vi "I(V)_MFLI_PK_v4.0_measureR.vi"() -> ()   [LabVIEW 2016]
uses:
  Labview Drivers/MFLI/LabOneLabVIEW-22.02.26577/LabOneLabVIEW-22.02.26577/Zurich Instruments LabOne/Public/Data/ziTypeDemodSampleSingle.ctl
  Labview Drivers/MFLI/LabOneLabVIEW-22.02.26577/LabOneLabVIEW-22.02.26577/Zurich Instruments LabOne/Public/Configure/ziSetValueDouble.vi
  Labview Drivers/MFLI/LabOneLabVIEW-22.02.26577/LabOneLabVIEW-22.02.26577/Zurich Instruments LabOne/Public/Configure/ziGetValueDemodSampleEx.vi
  Labview Drivers/MFLI/LabOneLabVIEW-22.02.26577/LabOneLabVIEW-22.02.26577/Zurich Instruments LabOne/Zurich Instruments LabOne.lvlib
panel:
  out "Set Voltage(V)":dbl format="%#_13g"
  out "Time(s)":dbl format="%#_13g"
  out "Demod Sample Out 2":T1={"Timestamps (ticks)"=34359738372, "X (Vrms)"=8.366245757779461e-285, "Y (Vrms)"=1.0096057436928657e-284, "Osc Phase (deg)"=1.69759663376e-313, "Freq (Hz)"=2.607691286315397e-191, "DIO"=4, "AuxIn0 (V)"=0.0, "AuxIn1 (V)"=1.6954746369817e-311, "Trigger"=16}
  out "Demod Sample Out":T1={"Timestamps (ticks)"=34359738372, "X (Vrms)"=8.366245757779461e-285, "Y (Vrms)"=1.0096057436928657e-284, "Osc Phase (deg)"=1.69759663376e-313, "Freq (Hz)"=2.607691286315397e-191, "DIO"=4, "AuxIn0 (V)"=0.0, "AuxIn1 (V)"=1.6954746369817e-311, "Trigger"=16}
  in  "MFLI Current source/Voltage reader":string="DEV4382"
  out "Imeas (A)":dbl=2.528615115e-315
  out "Vmeas (V)":dbl=nan
  in  "Folder":path=path "D:/Pranava/Data/Mn3Ge/MA1141"
  in  "wait (ms) [Should be > TC]":u32=1000
  out "I vs V":cluster{dbl, "Field Reading":dbl}[](graph)=[{nan, "Field Reading"=3.54694038e-315}, {nan, "Field Reading"=2.528615115e-315}]
  out "data":dbl[](array[numeric])=[nan, 2.528615115e-315, 0.0001]
  in  "Step":dbl[](array[numeric])=[0.05, 0.05, 0.05] min=-3000.0 max=3000.0 format="%.1e"
  in  "To":dbl[](array[numeric])=[7.0, -7.0, 0.0] min=-3000.0 max=3000.0 format="%.1e"
  in  "From":dbl[](array[numeric])=[0.0, 7.0, -7.0] min=-3000.0 max=3000.0 format="%.1e"
  in  "file name":string="002_MA1141_Mn3Ge(1120)IV_VdP_4K_slow"
  out "File path":path=path "D:/Pranava/Data/Mn3Ge/MA1141/002_MA1141_Mn3Ge(1120)IV_VdP_4K_slow.dat"
  # ".dat"
  # "Set MFLI Voltage output (V)"
types:
  T1 = typedef "Zurich Instruments LabOne.lvlib/ziTypeDemodSampleSingle.ctl" = cluster{"Timestamps (ticks)":u64, "X (Vrms)":dbl, "Y (Vrms)":dbl, "Osc Phase (deg)":dbl, "Freq (Hz)":dbl, "DIO":u32, "AuxIn0 (V)":dbl, "AuxIn1 (V)":dbl, "Trigger":u32}
  T2 = enum16{"open", "replace", "create", "open or create", "replace or create", "replace or create with confirmation"}
  T3 = typedef "Zurich Instruments LabOne.lvlib/ziTypeHandle.ctl" = cluster{"handleValid":bool, "Conn":u64, "Path Prefix":string, "Handle":u64, "Connected":bool, "Clockbase(s)":dbl}
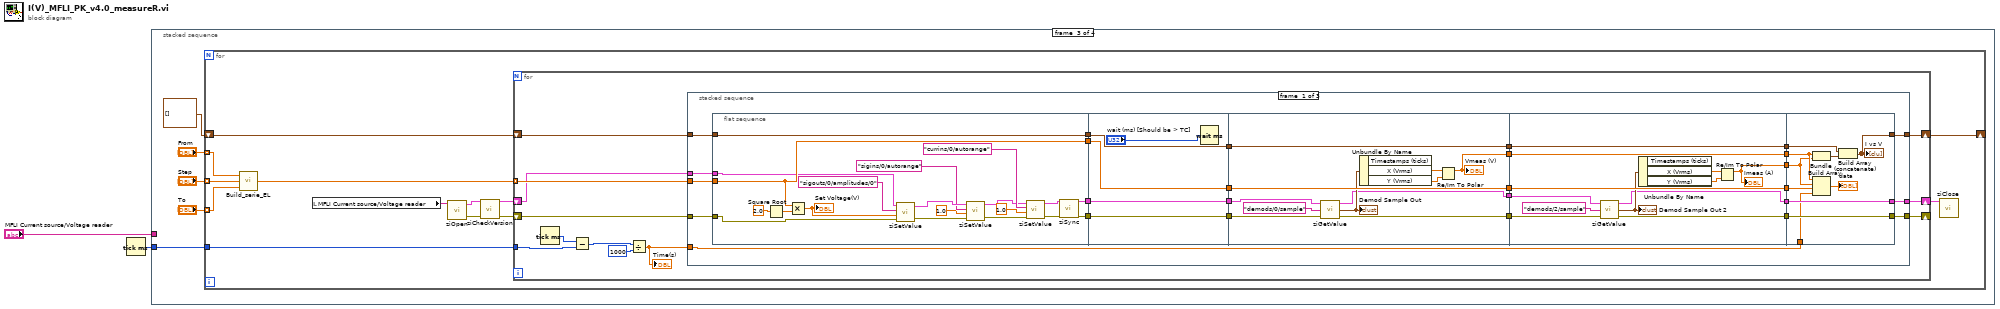
[diagram p0: block diagram]
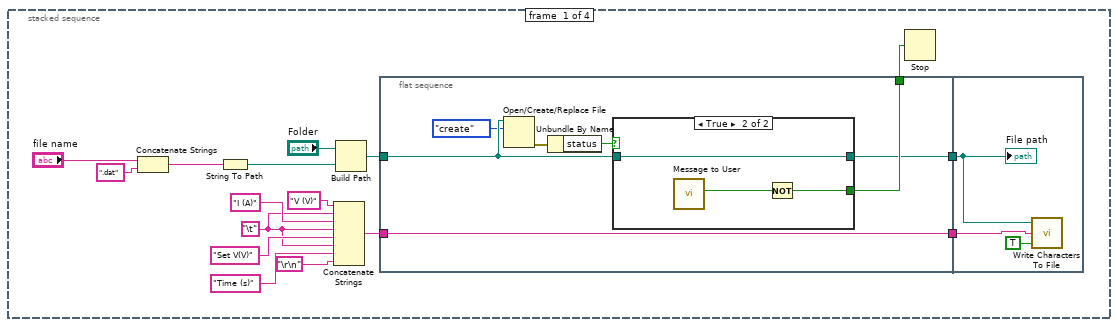
[diagram p2: hidden frame]
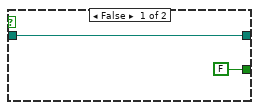
[diagram p3: hidden frame]
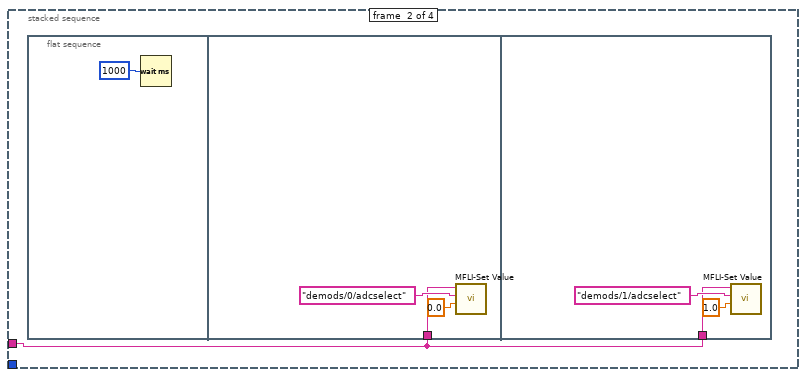
[diagram p4: hidden frame]
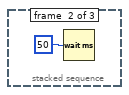
[diagram p5: hidden frame]
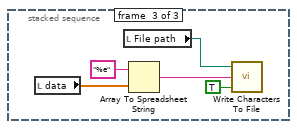
[diagram p6: hidden frame]
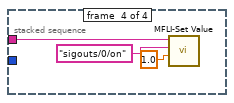
[diagram p7: hidden frame]
diagram:
  n1 = Tick Count (ms)() -> (millisecond timer value=w1:u32)
  n2 = stacked-sequence {
    tunnel: "MFLI Current source/Voltage reader" -> [_ w34 _ w163]
    tunnel: w1 -> [_ _ w42 _]
    frame #0 {
      w4 = "\t"
      n3 = Concatenate Strings("file name", ".dat" ("string")) -> (w15:string)
      n4 = String To Path(string=w15) -> (path=w7:path)
      n5 = Concatenate Strings("V (V)" ("string"), w4, "I (A)" ("string"), w4, "Set V(V)" ("string"), w4, "Time (s)", "\r\n") -> (w16:string)
      n6 = Build Path(base path="Folder", name or relative path=w7) -> (appended path=w6:path)
      n7 = flat-sequence {
        tunnel: w6 -> [w22]
        tunnel: w16 -> [w25]
        tunnel: [w25] -> w18
        tunnel: [w24] -> w13
        tunnel: [w23] -> w17
        tunnel: w18 -> [w32]
        tunnel: w17 -> [w31]
        frame #0 {
          n8 = Open/Create/Replace File(file path (use dialog)=w22, operation (0:open)=T2."create") -> (error out=w21:errorcluster)  [unwired: 4 in, 2 out]
          n9 = Unbundle By Name(w21) -> ("status"=w19:bool)
          n10 = case shown="True" w19 {
            tunnel: [FALSE ("Yes") w29] -> w24
            tunnel: [w26 w28] -> w23
            tunnel: w22 -> [w26 w28]
            frame False {
            }
            frame True {
              n11 = call "Message to User"() -> ("Yes"=w30:bool)  [unwired: 10 in, 1 out]
              n12 = Not(x=w30) -> (.not. x?=w29:bool)
            }
          }
        }
        frame #1 {
          n13 = call <vilib>:"Write Characters To File.vi"("append to file? (new file:F)"=TRUE, "character string"=w32, "file path (dialog if empty)"=w31) -> ()  [unwired: 2 in, 1 out]
          "File path" <- w31
        }
      }
      n14 = Stop(stop? (T)=w13) -> ()
    }
    frame #1 {
      n15 = flat-sequence {
        tunnel: w34 -> [w36]
        tunnel: w34 -> [w39]
        frame #0 {
          n16 = Wait (ms)(milliseconds to wait=u32 1000) -> ()  [unwired: 1 out]
        }
        frame #1 {
          n17 = call "MFLI-Set Value.vi"("Value"=0.0, "Path"="demods/0/adcselect", "MFLI Current source/Voltage reader"=w36) -> ()  [unwired: 9 in]
        }
        frame #2 {
          n18 = call "MFLI-Set Value.vi"("Value"=1.0, "Path"="demods/1/adcselect", "MFLI Current source/Voltage reader"=w39) -> ()  [unwired: 9 in]
        }
      }
    }
    frame #2 {
      n19 = for {
        tunnel: "From" -> [w56] mode=indexing
        tunnel: "To" -> [w55] mode=indexing
        tunnel: "Step" -> [w54] mode=indexing
        shift-right: [w58] -> _
        shift-left: cluster{dbl, "Field Reading":dbl}[] [] -> [w59]
        tunnel: w42 -> [w47]
        n20 = call "Build_serie_EL.vi"("end value"=w55, "increment"=w54, "start value"=w56) -> ("output array"=w57:dbl[])
        n21 = local read "MFLI Current source/Voltage reader"() -> (w53:string)
        n22 = call "ziOpen.vi"("Address"=w53) -> ("Error Out"=w52:errorcluster, "HandleOut"=w51:T3)  [unwired: 3 in, 1 out]
        n23 = call "ziCheckVersion.vi"("Handle In"=w51, "Error In"=w52) -> ("Handle Out"=w50:T3, "Error Out"=w48:errorcluster)  [unwired: 11 in, 1 out]
        n24 = for {
          tunnel: w57 -> [w71] mode=indexing
          shift-right: [w69] -> w58
          shift-left: w59 -> [w70]
          shift-right: [w66] -> w49
          shift-left: w50 -> [w68]
          shift-right: [w65] -> _
          shift-left: w48 -> [w67]
          tunnel: w47 -> [w61]
          n25 = Tick Count (ms)() -> (millisecond timer value=w62:u32)
          n26 = Subtract(x=w62, y=w61) -> (x-y=w63:u32)
          n27 = Divide(x=w63, y=1000) -> (x/y=w60:dbl)
          "Time(s)" <- w60
          n28 = stacked-sequence {
            tunnel: w71 -> [w96 _ _]
            tunnel: w70 -> [w97 _ _]
            tunnel: [w98 _ _] -> w69
            tunnel: w68 -> [w87 _ _]
            tunnel: w67 -> [w86 _ _]
            tunnel: [w76 _ _] -> w66
            tunnel: [w75 _ _] -> w65
            tunnel: w60 -> [w72 _ _]
            frame #0 {
              n29 = flat-sequence {
                tunnel: [w118] -> w93
                tunnel: [w117] -> w92
                tunnel: w96 -> [w117]
                tunnel: w97 -> [w118]
                tunnel: [w100] -> w89
                tunnel: [w101] -> w88
                tunnel: w87 -> [w103]
                tunnel: w86 -> [w102]
                tunnel: w93 -> [w123]
                tunnel: [w123] -> w95
                tunnel: w92 -> [w122]
                tunnel: [w122] -> w94
                tunnel: [w120] -> w91
                tunnel: [w119] -> w90
                tunnel: w89 -> [w119]
                tunnel: w88 -> [w120]
                tunnel: [w124] -> w85
                tunnel: [w134] -> w83
                tunnel: [w133] -> w81
                tunnel: w90 -> [w130]
                tunnel: w91 -> [w129]
                tunnel: w95 -> [w134]
                tunnel: w94 -> [w133]
                tunnel: [w128] -> w79
                tunnel: [w127] -> w78
                tunnel: w85 -> [w138]
                tunnel: [w138] -> w84
                tunnel: w83 -> [w146]
                tunnel: [w146] -> w82
                tunnel: w81 -> [w145]
                tunnel: [w145] -> w80
                tunnel: w79 -> [w142]
                tunnel: w78 -> [w141]
                tunnel: [w140] -> w77
                tunnel: [w139] -> w74
                tunnel: [w135] -> w73
                tunnel: w84 -> [w155]
                tunnel: [w154] -> w98
                tunnel: w82 -> [w153]
                tunnel: w80 -> [w152]
                tunnel: [w151] -> w76
                tunnel: w77 -> [w151]
                tunnel: [w150] -> w75
                tunnel: w74 -> [w150]
                tunnel: w73 -> [w149]
                tunnel: w72 -> [w147]
                frame #0 {
                  n30 = Square Root(x=2.0) -> (sqrt(x)=w116:dbl)
                  n31 = Multiply(x=w117, y=w116) -> (x*y=w99:dbl)
                  "Set Voltage(V)" <- w99
                  n32 = call-poly "ziSetValue.vi"("Error In"=w102, "Value"=w99, "Path"="sigouts/0/amplitudes/0", "Handle In"=w103) -> ("Error Out"=w110:errorcluster, "Handle Out"=w113:T3)  [unwired: 1 in]
                  n33 = call-poly "ziSetValue.vi"("Error In"=w110, "Value"=1.0, "Path"="sigins/0/autorange", "Handle In"=w113) -> ("Error Out"=w106:errorcluster, "Handle Out"=w107:T3)  [unwired: 1 in]
                  n34 = call-poly "ziSetValue.vi"("Error In"=w106, "Value"=1.0, "Path"="currins/0/autorange", "Handle In"=w107) -> ("Error Out"=w104:errorcluster, "Handle Out"=w105:T3)  [unwired: 1 in]
                  n35 = call "ziSync.vi"("Handle In"=w105, "Error In"=w104) -> ("Handle Out"=w101:T3, "Error Out"=w100:errorcluster)  [unwired: 12 in]
                }
                frame #1 {
                  n36 = Wait (ms)(milliseconds to wait="wait (ms) [Should be > TC]") -> ()  [unwired: 1 out]
                }
                frame #2 {
                  n37 = call-poly "ziGetValue.vi"("error in"=w130, "Path"="demods/0/sample", "Handle In"=w129) -> ("error out"=w127:errorcluster, "Demod Sample Out"=w131:T1, "Handle Out"=w128:T3)
                  "Demod Sample Out" <- w131
                  n38 = Unbundle By Name(w131) -> ("X (Vrms)"=w126:dbl, "Y (Vrms)"=w125:dbl)  [unwired: 1 out]
                  n39 = Re/Im To Polar(2:w125, 3:w126) -> (1:w124:dbl)  [unwired: 1 out]
                  "Vmeas (V)" <- w124
                }
                frame #3 {
                  n40 = call-poly "ziGetValue.vi"("error in"=w141, "Path"="demods/2/sample", "Handle In"=w142) -> ("error out"=w139:errorcluster, "Demod Sample Out"=w143:T1, "Handle Out"=w140:T3)
                  "Demod Sample Out 2" <- w143
                  n41 = Unbundle By Name(w143) -> ("X (Vrms)"=w136:dbl, "Y (Vrms)"=w137:dbl)  [unwired: 1 out]
                  n42 = Re/Im To Polar(2:w137, 3:w136) -> (1:w135:dbl)  [unwired: 1 out]
                  "Imeas (A)" <- w135
                }
                frame #4 {
                  n43 = Bundle(w155, w149) -> (w148:cluster{dbl, dbl})  [unwired: 1 in]
                  n44 = Build Array(w155, w149, w152, w147) -> (→"data":dbl[])
                  n45 = Build Array (concatenate)(w153, w148) -> (w154:cluster{dbl, "Field Reading":dbl}[])
                  "I vs V" <- w154
                }
              }
            }
            frame #1 {
              n46 = Wait (ms)(milliseconds to wait=u32 50) -> ()  [unwired: 1 out]
            }
            frame #2 {
              n47 = local read "data"() -> (w158:dbl[])
              n48 = local read "File path"() -> (w160:path)
              n49 = Array To Spreadsheet String(array=w158, 3:"%e" ("format string")) -> (spreadsheet string=w161:string)  [unwired: 1 in]
              n50 = call <vilib>:"Write Characters To File.vi"("append to file? (new file:F)"=TRUE, "character string"=w161, "file path (dialog if empty)"=w160) -> ()  [unwired: 2 in, 1 out]
            }
          }
        }
        n51 = call "ziClose.vi"("Handle In"=w49) -> ()  [unwired: 1 in, 4 out]
      }
    }
    frame #3 {
      n52 = call "MFLI-Set Value.vi"("Value"=1.0, "Path"="sigouts/0/on", "MFLI Current source/Voltage reader"=w163) -> ()  [unwired: 9 in]
    }
  }
